vi "Data.vi"(11 "Teardown Msg in":refnum<class "Teardown Msg.lvclass">) -> ()   [LabVIEW 2021, in "Teardown.lvlib" / "Teardown Msg.lvclass"]
uses:
  Teardown Msg.lvclass
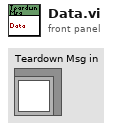
[diagram p1: front panel]
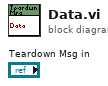
[diagram p0: block diagram]
diagram:
